vi "Update.vi"(8 "error in (no error)":errorcluster, 10 "Engine in":refnum<class "Engine.lvclass">, 11 "AttractScreen in":refnum<class "AttractScreen.lvclass">) -> (0 "error out":errorcluster, 2 "Engine out":refnum<class "Engine.lvclass">, 3 "AttractScreen out":refnum<class "AttractScreen.lvclass">)   [LabVIEW 2019, in "RT_Game.lvlib" / "AttractScreen.lvclass"]
uses:
  AttractScreen.lvclass
  C:/Users/FreshBob/Dropbox/VIs/myRIO_GameConsole/RT/RT_Game/Game/Game.lvclass
  Engine/Engine.lvclass
  Game/Game.lvclass/Game.ctl
  AttractScreen.lvclass/AttractScreen.ctl
  AttractStates.ctl
  Game/Read State.vi
  Engine/Globals.vi
  Game/Game.lvclass
  FadeOutTiles/FadeOutTiles.lvclass
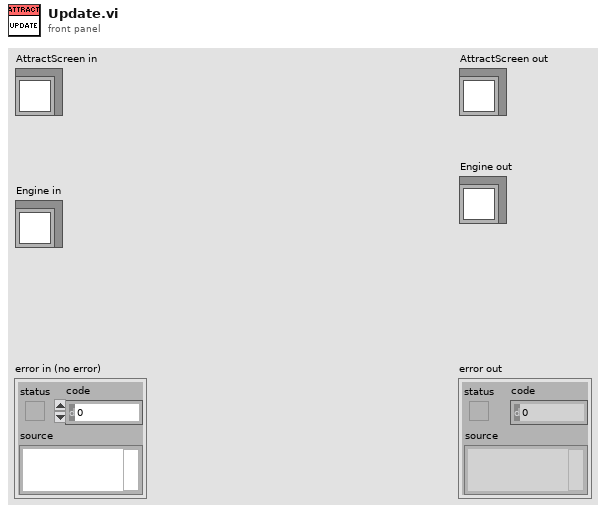
[diagram p1: front panel]
types:
  T1 = typedef "RT_Game.lvlib/Game.lvclass/States.ctl" = enum16{"Init", "Restart", "Menu", "Game", "Resume", "ToggleSingleplayer", "LoadNextGame", "ExitToMenu", "NewHighscore", "GameOver", "SlideOut", "FadeToMenu", "StartFadeToMenu"}
  T2 = typedef "RT_Game.lvlib/AttractScreen.lvclass/AttractStates.ctl" = enum16{"FadeIn", "Display", "FadeOut"}
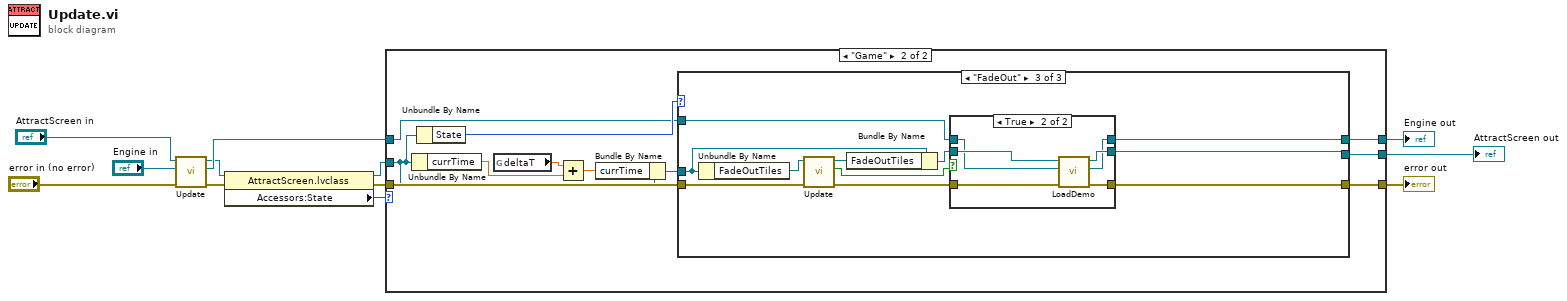
[diagram p0: block diagram]
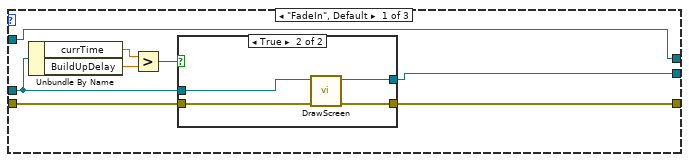
[diagram p3: hidden frame]
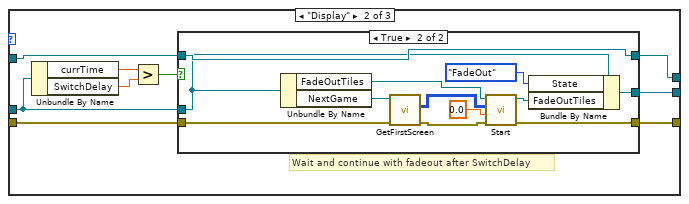
[diagram p5: hidden frame]
diagram:
  n1 = call-parent "Update.vi"("error in (no error)"="error in (no error)", "Engine in"="Engine in", "Game in"="AttractScreen in") -> ("error out"=w9:errorcluster, "Engine out"=w8:refnum<class "Engine.lvclass">, "Game out"=w3:refnum<class "AttractScreen.lvclass">)  [unwired: 6 in]
  n2 = property class="AttractScreen.lvclass"(reference=w3, error in=w9) -> (reference out=w2:refnum<class "AttractScreen.lvclass">, error out=w4:errorcluster, "Accessors:State"=w1:T1)
  n3 = case shown="\"Game\"" w1 {
    tunnel: w4 -> [w13 w25]
    tunnel: w8 -> [w15 w24]
    tunnel: w2 -> [w14 w23]
    tunnel: [w13 w18] -> w7
    tunnel: [w14 w17] -> w6
    tunnel: [w15 w16] -> w5
    frame "Init", Default {
    }
    frame "Game" {
      n4 = Unbundle By Name(w23) -> ("currTime"=w21:dbl)
      n5 = Unbundle By Name(w23) -> ("State"=w26:T2)
      n6 = global read "Globals.vi" "deltaT"() -> (w19:dbl)
      n7 = Add(x=w19, y=w21) -> (x+y=w20:dbl)
      n8 = Bundle By Name(cluster=w23, "currTime"=w20) -> (w22:refnum<class "AttractScreen.lvclass">)
      n9 = case shown="\"FadeOut\"" w26 {
        tunnel: w22 -> [w31 w42 w70]
        tunnel: w25 -> [w34 w49 w75]
        tunnel: [w33 w47 w73] -> w17
        tunnel: [w32 w48 w74] -> w18
        tunnel: w24 -> [w27 w46 w72]
        tunnel: [w27 w45 w71] -> w16
        frame "FadeIn", Default {
          n10 = Unbundle By Name(w31) -> ("currTime"=w29:dbl, "BuildUpDelay"=w30:dbl)
          n11 = Greater?(x=w29, y=w30) -> (0:w28:bool)
          n12 = case shown="True" w28 {
            tunnel: w31 -> [w36 w40]
            tunnel: w34 -> [w35 w39]
            tunnel: [w36 w38] -> w33
            tunnel: [w35 w37] -> w32
            frame False {
            }
            frame True {
              n13 = call "DrawScreen.vi"("error in (no error)"=w39, "AttractScreen in"=w40) -> ("error out"=w37:errorcluster, "AttractScreen out"=w38:refnum<class "AttractScreen.lvclass">)  [unwired: 8 in]
            }
          }
        }
        frame "Display" {
          # "Wait and continue with fadeout after SwitchDelay"
          n14 = Unbundle By Name(w42) -> ("currTime"=w43:dbl, "SwitchDelay"=w44:dbl)
          n15 = Greater?(x=w43, y=w44) -> (0:w41:bool)
          n16 = case shown="True" w41 {
            tunnel: w49 -> [w51 w63]
            tunnel: [w51 w59] -> w48
            tunnel: w42 -> [w52 w60]
            tunnel: [w52 w62] -> w47
            tunnel: w46 -> [w50 w64]
            tunnel: [w50 w64] -> w45
            frame False {
            }
            frame True {
              n17 = Unbundle By Name(w60) -> ("FadeOutTiles"=w58:refnum<class "FadeOutTiles.lvclass">, "NextGame"=w55:refnum<class "Game.lvclass">)
              n18 = call-dynamic "GetFirstScreen.vi"("error in (no error)"=w63, "Game in"=w55) -> ("error out"=w56:errorcluster, "Array"=w54:u32[][])  [unwired: 7 in, 1 out]
              n19 = call "Start.vi"("error in (no error)"=w56, "FadeRate"=0.0, "FadePicture"=w54, "FadeOutTiles in"=w58) -> ("error out"=w59:errorcluster, "FadeOutTiles out"=w57:refnum<class "FadeOutTiles.lvclass">)  [unwired: 6 in]
              n20 = Bundle By Name(cluster=w60, "State"=AttractStates."FadeOut", "FadeOutTiles"=w57) -> (w62:refnum<class "AttractScreen.lvclass">)
            }
          }
        }
        frame "FadeOut" {
          n21 = Unbundle By Name(w70) -> ("FadeOutTiles"=w67:refnum<class "FadeOutTiles.lvclass">)
          n22 = call "Update.vi"("error in (no error)"=w75, "FadeOutTiles in"=w67) -> ("error out"=w68:errorcluster, "Done?"=w65:bool, "FadeOutTiles out"=w66:refnum<class "FadeOutTiles.lvclass">)  [unwired: 7 in]
          n23 = Bundle By Name(cluster=w70, "FadeOutTiles"=w66) -> (w69:refnum<class "AttractScreen.lvclass">)
          n24 = case shown="True" w65 {
            tunnel: w68 -> [w76 w84]
            tunnel: [w76 w83] -> w74
            tunnel: w69 -> [w77 w82]
            tunnel: [w77 w81] -> w73
            tunnel: w72 -> [w78 w80]
            tunnel: [w78 w79] -> w71
            frame False {
            }
            frame True {
              n25 = call "LoadDemo.vi"("error in (no error)"=w84, "Engine in"=w80, "AttractScreen in"=w82) -> ("error out"=w83:errorcluster, "Engine out"=w79:refnum<class "Engine.lvclass">, "AttractScreen out"=w81:refnum<class "AttractScreen.lvclass">)  [unwired: 6 in]
            }
          }
        }
      }
    }
  }
  "error out" <- w7
  "AttractScreen out" <- w6
  "Engine out" <- w5
